vi "test_GetItemInformationFromProjects_SplitProjectTargetsSolution.vi"() -> (3 "Pass?":bool)   [LabVIEW 2019, in "Tests.SolutionBuilder.lvlib"]
uses:
  Tests.SolutionBuilder.lvlib
  SolutionBuilder/SolutionBuilder.lvclass
  SolutionBuilder/ProjectItem/ProjectItem.lvclass
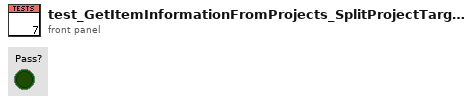
[diagram p1: front panel]
types:
  T1 = cluster{"Relative Path from 1 to 2":path, string[]}
  T2 = cluster{"Relative Path from 1 to 2":path, string[]}[]
  T3 = typedef "SolutionBuilder.lvlib/SolutionBuilder.lvclass/ProjectItemMap.ctl" = map{path, refnum<class "ProjectItem.lvclass">[]}
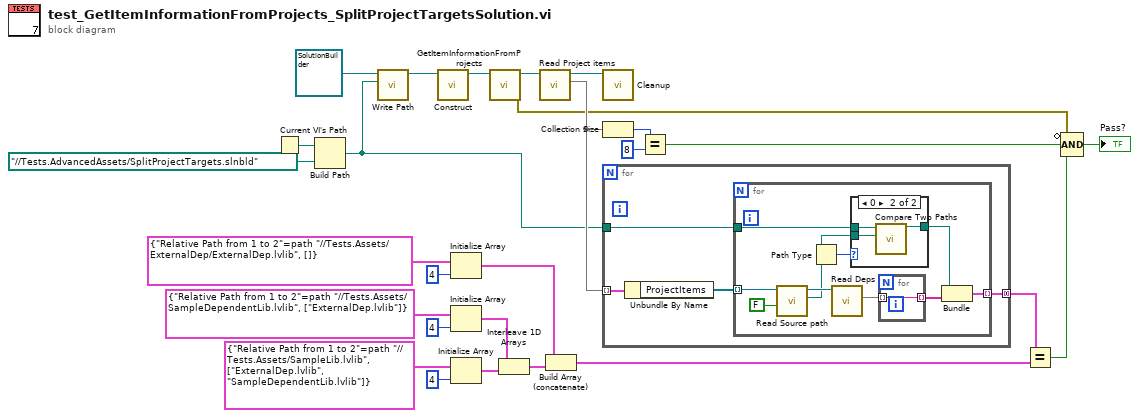
[diagram p0: block diagram]
diagram:
  n1 = Current VI's Path() -> (path=w26:path)
  n2 = Build Path(base path=w26, name or relative path=path "../../Tests.AdvancedAssets/SplitProjectTargets.slnbld" ("Path")) -> (appended path=w14:path)
  n3 = call "Write Path.vi"("Path"=w14, "SolutionBuilder in"=refnum<class "SolutionBuilder.lvclass"> refnum) -> ("SolutionBuilder out"=w20:refnum<class "SolutionBuilder.lvclass">)  [unwired: 9 in]
  n4 = call "Construct.vi"("SolutionBuilder in"=w20) -> ("SolutionBuilder out"=w17:refnum<class "SolutionBuilder.lvclass">)  [unwired: 9 in, 1 out]
  n5 = Initialize Array(T1 {"Relative Path from 1 to 2"=path "../../Tests.Assets/ExternalDep/ExternalDep.lvlib", []}, 4 ("dimension size")) -> (w4:T2)
  n6 = Initialize Array(T1 {"Relative Path from 1 to 2"=path "../../Tests.Assets/SampleDependentLib.lvlib", ["ExternalDep.lvlib"]}, 4 ("dimension size")) -> (w6:T2)
  n7 = Initialize Array(T1 {"Relative Path from 1 to 2"=path "../../Tests.Assets/SampleLib.lvlib", ["ExternalDep.lvlib", "SampleDependentLib.lvlib"]}, 4 ("dimension size")) -> (w5:T2)
  n8 = call "GetItemInformationFromProjects.vi"("SolutionBuilder in"=w17) -> ("error out"=w13:errorcluster, "SolutionBuilder out"=w16:refnum<class "SolutionBuilder.lvclass">)  [unwired: 9 in]
  n9 = Interleave 1D Arrays(w6, w5) -> (w3:T2)
  n10 = call "Read Project items.vi"("SolutionBuilder in"=w16) -> ("Project items"=w22:T3, "SolutionBuilder out"=w19:refnum<class "SolutionBuilder.lvclass">)  [unwired: 9 in]
  n11 = Build Array (concatenate)(w4, w3) -> (w2:T2)
  n12 = call "Cleanup.vi"("SolutionBuilder in"=w19) -> ()  [unwired: 9 in, 2 out]
  n13 = Collection Size(1:w22) -> (0:w24:i32)
  n14 = for {
    tunnel: w22 -> [w31] mode=indexing
    tunnel: [w29] -> w15 mode=concatenating
    tunnel: w14 -> [w28]
    n15 = Unbundle By Name(w31) -> ("ProjectItems"=w30:refnum<class "ProjectItem.lvclass">[])
    n16 = for {
      tunnel: w30 -> [w38] mode=indexing
      tunnel: [w39] -> w29 mode=indexing
      tunnel: w28 -> [w32]
      n17 = call "Read Source path.vi"("Force abs path? (T)"=FALSE, "ProjectItem in"=w38) -> ("Source path"=w33:path, "ProjectItem out"=w37:refnum<class "ProjectItem.lvclass">)  [unwired: 8 in]
      n18 = Path Type(1:w33) -> (0:w35:i16)
      n19 = call "Read Deps.vi"("ProjectItem in"=w37) -> ("Deps"=w41:set{string})  [unwired: 9 in, 1 out]
      n20 = case shown="0" w35 {
        tunnel: w33 -> [w42 w43]
        tunnel: [w42 w45] -> w34
        tunnel: w32 -> [_ w44]
        frame Default {
        }
        frame 0 {
          n21 = call <vilib>:"Compare Two Paths.vi"("Path 2"=w43, "Path 1"=w44) -> ("Relative Path from 1 to 2"=w45:path)  [unwired: 6 in, 3 out]
        }
      }
      n22 = for {
        tunnel: w41 -> [w46] mode=indexing
        tunnel: [w46] -> w40 mode=indexing
      }
      n23 = Bundle("Relative Path from 1 to 2"=w34, w40) -> (w39:T1)  [unwired: 1 in]
    }
  }
  n24 = Equal?(x=w24, y=8) -> (x = y?=w21:bool)
  n25 = Equal?(x=w15, y=w2) -> (x = y?=w18:bool)
  n26 = Compound Arithmetic op=AND(invert w13, w21, w18) -> (→"Pass?":bool)
